vi "UHR-Fleezers Control (host) -Mau_stepping_gamma.vi"(0 "Tab Control":T5(tab)) -> ()   [LabVIEW 2013] (continued)
  n71 = local write "Update Count (MCL)"(w101) -> ()
  n72 = local write "Total Counts (ticks)"(w101) -> ()
  n73 = xnode "Invoke Method"("FPGA VI Reference In"=w218) -> ("FPGA VI Reference Out"=w120:T19, "error out"=w139:errorcluster)  [unwired: 1 in]
  n74 = local write "Ave. Period (s)"(w170) -> ()
  n75 = property on="2D or 1D Scan" class="Bool (strict)"("Val(Sgnl)"=w122) -> ()  [unwired: 2 in, 2 out]
  n76 = xnode "Read/Write Control"("FPGA VI Reference In"=w119, "error in"=w139, "ai count"="AI Count (ticks)", "Interlace ON/OFF"=w104, "Number Interlace Cycles"=w103, "AI1 Sets to FIFO"=w233, "FB On/Off Set 1"=w232, "FB On/Off Set 2"=w231, "Interlace Off Parameters"=w102, "FB Setpoint Set 1"=w223, "FB Setpoint Set 2"=w222, "FB Gains Set 1"=w220, "FB Gains Set 2"=w219, "FB output range 1"=w121, "FB output range 2"=w121, "Cycles per step"=w204, "Scan BD"=w216, "Number of scans"=w200, "Scan steps"=w205, "Scan freq.  increment"=w206, "AO1"=w188, "AO2"=w187, "Scan freq.  increment (MCL)"=w181, "Scan steps (MCL)"=w180, "Cycles per step (MCL)"=w179, "Number of scans (MCL)"=w178, "MCL count"=w101, "Cont. Scan (MCL)"=w177, "MCL Scan Axis"=w171, "1D or 2D Scan?"=w122, "N of AI1 Int Acq Sets"=w161, "Freq or Amp switch first"="Freq or Amp switch first", "Freq switch delay"="Freq switch delay", "Amp switch delay"="Amp switch delay", "Swap F1 and F2"="Swap F1 and F2", "APD Acq Rate Count"=w127, "APD to FIFO"=FALSE, "APD Gate Operating Mode"="APD Gate", "APD Gate ON Count"="APD Gate ON Count", "APD Gate OFF Count"="APD Gate OFF Count", "Invert APD Gate"="Invert APD Gate", "DIO count 1 (ticks)"="DIO count 1 (ticks)", "DIO count 2 (ticks)"="DIO count 2 (ticks)", "DIO count 3 (ticks)"="DIO count 3 (ticks)", "APD 1 AO scale factor"="APD 1 AO Mult.", "APD 2 AO scale factor"="APD 2 AO Mult.") -> ("FPGA VI Reference Out"=w96:T19, "error out"=w98:errorcluster)  [unwired: 1 in]
  n77 = local read "Green Laser ON/Interlacing"() -> (w99:bool)
  n78 = local read "Green laser mode"() -> (w100:enum32{"Laser ON", "Laser OFF", "Interlace"})
  n79 = local read "GI Frequency, OFF count"() -> (w92:u32)
  n80 = local read "GI Frequency, ON count"() -> (w91:u32)
  n81 = Multiply(x="Current When FB OFF (%)", y=655.35) -> (x*y=w82:dbl)
  n82 = local read "Green FB Count"() -> (w90:u32)
  n83 = Multiply(x="Green FB Setpoint (mV)", y=3.2767) -> (x*y=w79:dbl)
  n84 = To Unsigned Word Integer(number=w82) -> (unsigned 16bit integer=w80:u16)
  n85 = local read "Invert GI"() -> (w94:bool)
  n86 = To Word Integer(number=w79) -> (16bit integer=w77:i16)
  n87 = case shown="True" w99 {
    tunnel: w100 -> [_ w253]
    tunnel: [enum32{"Laser ON", "Laser OFF", "Interlace"}."Laser OFF" ("Green laser mode") w253] -> w93
    frame False {
    }
    frame True {
    }
  }
  n88 = local read "Trap Pos. AI1 X Pre-scale"() -> (w48:u16)
  n89 = local read "Trap Pos FB Monitor\nT1 or T2"() -> (w55:bool)
  n90 = local read "Trap Pos FB Int Count"() -> (w43:u16)
  n91 = local read "Trap Pos FB Negate Action"() -> (w54:bool)
  n92 = local read "Trap Pos. FB Offset Factor"() -> (w53:i64)
  n93 = local read "Trap Pos. FB Mult Factor"() -> (w52:i64)
  n94 = local read "Trap Pos. FB Gains"() -> (w50:T11)
  n95 = local read "Trap Pos. FB Range"() -> (w51:T12)
  n96 = xnode "Read/Write Control"("FPGA VI Reference In"=w96, "error in"=w98, "Green interlace ON count 2"=w91, "Green interlace OFF count 2"=w92, "Invert GI 2"=w94, "Operating Mode 2"=w93, "Green FB Gains"="Green FB Gains", "Green FB Setpoint"=w77, "Green FB On/Off"="Green FB On/Off", "Current Out"=w80, "Green int current ON count adj"="Green int current ON count adj", "Green FB Count"=w90, "Operating Mode"=w93, "Green interlace OFF count"=w92, "Green interlace ON count"=w91, "Invert GI"=w94, "Trap Pos FB Monitor T1 or T2"=w55, "Trap Pos FB Negate Action"=w54, "Trap Pos. FB Offset Factor"=w53, "Trap Pos. FB Mult Factor"=w52, "Trap Pos. FB Range"=w51, "Trap Pos. FB Gains"=w50, "Force feedback"=FALSE, "AI1 X Scale"=w48, "Trap Pos to FIFO"=TRUE, "Trap Pos FB Int Count"=w43) -> ("FPGA VI Reference Out"=w95:T19, "error out"=w97:errorcluster)
  n97 = xnode "Invoke Method"("FPGA VI Reference In"=w95, "error in"=w97, "Requested Depth"="Trap AI FIFO Depth") -> ("FPGA VI Reference Out"=w58:T19, "error out"=w57:errorcluster)  [unwired: 1 out]
  n98 = xnode "Invoke Method"("FPGA VI Reference In"=w58, "error in"=w57, "Requested Depth"="Trap Position FIFO Depth") -> ("FPGA VI Reference Out"=w45:T19, "error out"=w44:errorcluster)  [unwired: 1 out]
  n99 = flat-sequence {
    tunnel: w120 -> [w258]
    tunnel: [w258] -> w119
    tunnel: [w257] -> w118
    tunnel: [w256] -> w117
    tunnel: [w254] -> w115
    tunnel: [w255] -> w116
    frame #0 {
      w255 = T16 {"Minimum"=50.0, "Maximum"=100.0, "Increment"=1.0} ("Min Max Inc")
      w254 = T16 {"Minimum"=0.0, "Maximum"=75.0, "Increment"=1.0} ("Data Entry Limits")
      w257 = T16 {"Minimum"=50.0, "Maximum"=100.0, "Increment"=1.0} ("Min Max Inc")
      w256 = T16 {"Minimum"=0.0, "Maximum"=75.0, "Increment"=1.0} ("Data Entry Limits")
      n100 = property on="BD 2 Frequency 1 (MHz)" class="DigNum (strict)"("Data Range"=w255) -> ()  [unwired: 2 in, 2 out]
      n101 = property on="BD 2 Frequency 3 (MHz)" class="DigNum (strict)"("Data Range"=w255) -> ()  [unwired: 2 in, 2 out]
      n102 = property on="BD 2 Frequency 2 (MHz)" class="DigNum (strict)"("Data Range"=w255) -> ()  [unwired: 2 in, 2 out]
      n103 = property on="BD 1 Frequency 1 (MHz)" class="DigNum (strict)"("Data Range"=w257) -> ()  [unwired: 2 in, 2 out]
      n104 = property on="BD 1 Frequency 2 (MHz)" class="DigNum (strict)"("Data Range"=w257) -> ()  [unwired: 2 in, 2 out]
      n105 = property on="BD 1 Frequency 3 (MHz)" class="DigNum (strict)"("Data Range"=w257) -> ()  [unwired: 2 in, 2 out]
      n106 = property on="BD 2 Amplitude 1 (%)" class="DigNum (strict)"("Data Range"=w254) -> ()  [unwired: 2 in, 2 out]
      n107 = property on="BD 2 Amplitude 2 (%)" class="DigNum (strict)"("Data Range"=w254) -> ()  [unwired: 2 in, 2 out]
      n108 = property on="BD 2 Amplitude 3 (%)" class="DigNum (strict)"("Data Range"=w254) -> ()  [unwired: 2 in, 2 out]
      n109 = property on="BD 1 Amplitude 3 (%)" class="DigNum (strict)"("Data Range"=w256) -> ()  [unwired: 2 in, 2 out]
      n110 = property on="BD 1 Amplitude 2 (%)" class="DigNum (strict)"("Data Range"=w256) -> ()  [unwired: 2 in, 2 out]
      n111 = property on="BD 1 Amplitude 1 (%)" class="DigNum (strict)"("Data Range"=w256) -> ()  [unwired: 2 in, 2 out]
      "X RF Frequency Limits (MHz)" <- w257
      "X RF Amplitude Limits (%)" <- w256
      "Y RF Amplitude Limits (%)" <- w254
      "Y RF Frequency Limits (MHz)" <- w255
    }
  }
  n112 = xnode "Invoke Method"("FPGA VI Reference In"=w45, "error in"=w44) -> ("FPGA VI Reference Out"=w22:T19, "error out"=w21:errorcluster)  [unwired: 1 in]
  n113 = flat-sequence "Initial FPGA Loop Relative Phase Adjustment" {
    tunnel: "Initial Phase Adjustment (APD 2 Gate)" -> [w260]
    tunnel: "Initial Phase Adjustment (GI) 2" -> [w261]
    tunnel: "Initial Phase Adj. (MCL)" -> [w262]
    tunnel: w21 -> [w263]
    tunnel: w22 -> [w264]
    tunnel: "Initial Phase Adjustment (GI)" -> [w265]
    tunnel: "Initial Phase Adjustment (AI1)" -> [w266]
    tunnel: [w266] -> w31
    tunnel: [w265] -> w30
    tunnel: [w264] -> w29
    tunnel: [w263] -> w28
    tunnel: [w262] -> w27
    tunnel: [w261] -> w26
    tunnel: [w260] -> w25
    tunnel: [w278] -> w145
    tunnel: [w272] -> w143
    tunnel: "Initial Phase Adjustment (APD Acq)" -> [w271]
    tunnel: "Initial Phase Adjustment (APD 1 Gate)" -> [w270]
    tunnel: "Initial Phase Adjustment (Green FB)" -> [w269]
    tunnel: w31 -> [w277]
    tunnel: w30 -> [w276]
    tunnel: w29 -> [w275]
    tunnel: w28 -> [w274]
    tunnel: w27 -> [w273]
    tunnel: w26 -> [w268]
    tunnel: w25 -> [w267]
    tunnel: w145 -> [w280]
    tunnel: [w281] -> w144
    tunnel: w143 -> [w281]
    tunnel: [w280] -> w142
    tunnel: w144 -> [w284]
    tunnel: w142 -> [w283]
    tunnel: [w286] -> w141
    tunnel: [w285] -> w140
    tunnel: [w288] -> w20
    tunnel: [w289] -> w23
    tunnel: w141 -> [w289]
    tunnel: w140 -> [w288]
    frame #0 {
      n114 = Wait (ms)(milliseconds to wait=u32 1000) -> ()  [unwired: 1 out]
    }
    frame #1 {
      n115 = xnode "Read/Write Control"("FPGA VI Reference In"=w275, "error in"=w274, "Phase count adjustment"=w277, "Phase count adjustment (GI)"=w276, "Phase count adjustment (MCL)"=w273, "Phase Count Adjustment (APD Acq)"=w271, "Phase count adjustment (APD 1 Gate)"=w270, "Phase count adjustment (APD 2 Gate)"=w267, "Phase count adjustment (Green FB)"=w269, "Phase count adjustment (GI) 2"=w268) -> ("FPGA VI Reference Out"=w272:T19, "error out"=w278:errorcluster)
    }
    frame #2 {
      n116 = Wait (ms)(milliseconds to wait=u32 1000) -> ()  [unwired: 1 out]
    }
    frame #3 {
      w282 = TRUE
      n117 = xnode "Read/Write Control"("FPGA VI Reference In"=w284, "error in"=w283, "+ phase"=w282, "+ phase (GI)"=w282, "+ phase (MCL)"=w282, "+ phase (APD Acq)"=w282, "+ phase (APD 1 Gate)"=w282, "+ phase (APD 2 Gate)"=w282, "+ phase (Green FB)"=w282, "+ phase (GI) 2"=w282) -> ("FPGA VI Reference Out"=w285:T19, "error out"=w286:errorcluster)
    }
    frame #4 {
      n118 = Wait (ms)(milliseconds to wait=u32 1000) -> ()  [unwired: 1 out]
    }
  }
  n119 = local read "Phase adj. (Green FB)"() -> (w113:i16)
  n120 = local read "Phase adj. (GI) 2"() -> (w83:i16)
  n121 = local read "Phase adjust (MCL)"() -> (w172:i16)
  n122 = local read "Phase adj. (AI1)"() -> (w174:i16)
  n123 = local read "Phase adj. (GI)"() -> (w173:i16)
  n124 = xnode "Read/Write Control"("FPGA VI Reference In"=w20, "error in"=w23, "Phase count adjustment"=w174, "Phase count adjustment (GI)"=w173, "Phase count adjustment (MCL)"=w172, "Phase Count Adjustment (APD Acq)"="Phase Adj. (APD Acq)", "Phase count adjustment (APD 1 Gate)"="Phase Adj. (APD 1 Gate)", "Phase count adjustment (APD 2 Gate)"="Phase Adj. (APD 2 Gate)", "Phase count adjustment (Green FB)"=w113, "Phase count adjustment (GI) 2"=w83) -> ("FPGA VI Reference Out"=w19:T19, "error out"=w18:errorcluster)
  n125 = call "Initialize RF boards - interlace 3.vi"("error in"=w18, "FPGA VI Reference In"=w19) -> ("FPGA VI Reference Out"=w150:T19)  [unwired: 1 out]
  n126 = call "set RF board frequency - interlace.vi"("Board 2 Frequency Limits"=w116, "Board 1 Frequency Limits"=w118, "FPGA VI Reference In"=w150, "Board 2 Frequency 3 (MHz)"="BD 2 Frequency 3 (MHz)", "Board 1 Frequency 3 (MHz)"="BD 1 Frequency 3 (MHz)", "Board 2 Frequency 2 (MHz)"="BD 2 Frequency 2 (MHz)", "Board 2 Frequency 1 (MHz)"="BD 2 Frequency 1 (MHz)", "Board 1 Frequency 2 (MHz)"="BD 1 Frequency 2 (MHz)", "Board 1 Frequency 1  (MHz)"="BD 1 Frequency 1 (MHz)") -> ("error out"=w244:errorcluster, "FPGA VI Reference Out"=w245:T19)  [unwired: 1 in]
  n127 = call "set RF board amplitude - interlace.vi"("Board 2 Amplitude Limits"=w115, "Board 1 Amplitude Limits"=w117, "error in"=w244, "FPGA VI Reference In"=w245, "Board 2 Amplitude 3 (%)"="BD 2 Amplitude 3 (%)", "Board 1 Amplitude 3 (%)"="BD 1 Amplitude 3 (%)", "Board 2 Amplitude 2 (%)"="BD 2 Amplitude 2 (%)", "Board 2 Amplitude 1 (%)"="BD 2 Amplitude 1 (%)", "Board 1 Amplitude 2 (%)"="BD 1 Amplitude 2 (%)", "Board 1 Amplitude 1 (%)"="BD 1 Amplitude 1 (%)") -> ("error out"=w16:errorcluster, "FPGA VI Reference Out"=w17:T19)
  n128 = flat-sequence {
    tunnel: w17 -> [w298]
    tunnel: w16 -> [w297]
    tunnel: [w296] -> w237
    tunnel: [w295] -> w236
    tunnel: [w302] -> w235
    tunnel: w237 -> [w302]
    tunnel: [w301] -> w234
    tunnel: w236 -> [w301]
    tunnel: w235 -> [w311]
    tunnel: w234 -> [w310]
    tunnel: [w309] -> w12
    tunnel: [w304] -> w11
    tunnel: [w314] -> w40
    tunnel: [w318] -> w24
    tunnel: w12 -> [w318]
    tunnel: w11 -> [w313]
    frame #0 {
      n129 = local read "Trap 1 (ON/OFF)"() -> (w290:bool)
      n130 = xnode "Read/Write Control"("FPGA VI Reference In"=w298, "error in"=w297, "Direct RF Box  Communication"=FALSE) -> ("FPGA VI Reference Out"=w296:T19, "error out"=w295:errorcluster)
      n131 = local write "Saving..."(FALSE ("Saving Data")) -> ()
      n132 = local write "Stop All"(FALSE ("Stop All")) -> ()
      n133 = local write "Index"(1.0 ("Index")) -> ()
      n134 = property on="Trap 1 ON" class="Bool (strict)"("Value"=w290) -> ()  [unwired: 2 in, 2 out]
      "Manipulating Trap" <- FALSE ("Manipulating Trap")
    }
    frame #1 {
      n135 = local read "Trap 2 (ON/OFF)"() -> (w300:bool)
      n136 = Wait (ms)(milliseconds to wait=u32 50) -> ()  [unwired: 1 out]
      n137 = property on="Trap 2 ON" class="Bool (strict)"("Val(Sgnl)"=w300) -> ()  [unwired: 2 in, 2 out]
    }
    frame #2 {
      n138 = local read "Scan Range (nm)"() -> (w305:dbl)
      n139 = xnode "Read/Write Control"("FPGA VI Reference In"=w311, "error in"=w310, "FPGA Controls  RF Box"=TRUE ("Direct RF Box  Communication")) -> ("FPGA VI Reference Out"=w309:T19, "error out"=w304:errorcluster)
      n140 = call "Update messages.vi"("Message to add"="UHR-Fleezers ready.", "Old message string"="") -> ("New message string"=w308:string)
      n141 = local write "Messages"(w308) -> ()
      n142 = property on="Scan Range (nm)" class="DigNum (strict)"("Val(Sgnl)"=w305) -> ()  [unwired: 2 in, 2 out]
    }
    frame #3 {
      n143 = call "hamilton_controller.vi"("error in"=w313, "action"=T20."CONNECT") -> ("error out"=w315:errorcluster)  [unwired: 9 in]
      n144 = call "hamilton_controller.vi"("error in"=w315, "action"=T20."INITIALIZE VALVES") -> ("error out"=w314:errorcluster)  [unwired: 9 in]
    }
  }
  n145 = Subtract(x="BD 1 Frequency 1 (MHz)", y="BD 1 Frequency 2 (MHz)") -> (x-y=w160:dbl)
  n146 = Subtract(x="BD 2 Frequency 1 (MHz)", y="BD 2 Frequency 2 (MHz)") -> (x-y=w159:dbl)
  n147 = Square(x=w159) -> (x^2=w157:dbl)
  n148 = Square(x=w160) -> (x^2=w158:dbl)
  n149 = Add(x=w158, y=w157) -> (x+y=w156:dbl)
  n150 = Square Root(x=w156) -> (sqrt(x)=w155:dbl)
  n151 = local write "Trap Delta (MHz)"(w155) -> ()
  n152 = call "IMAQ Create"("Image Name"="APD 1 Image", "Image Type"=w64) -> ("New Image"=w63:T3)  [unwired: 3 in, 1 out]
  n153 = call "IMAQ Create"("Image Name"="APD 2 Image", "Image Type"=w64) -> ("New Image"=w62:T3)  [unwired: 3 in, 1 out]
  n154 = call "IMAQ Create"("Image Name"="Det. X Image", "Image Type"=w64) -> ("New Image"=w61:T3)  [unwired: 3 in, 1 out]
  n155 = call "IMAQ Create"("Image Name"="Det. Y Image", "Image Type"=w64) -> ("New Image"=w60:T3)  [unwired: 3 in, 1 out]
  n156 = Bundle("New Image"=w63, "New Image"=w62, "New Image"=w61, "New Image"=w60) -> (w59:T21)  [unwired: 1 in]
  n157 = Current VI's Path() -> (path=w1:path)
  n158 = Concatenate Strings("N.D.", "\r\n") -> (w5:string)
  n159 = Strip Path(path=w1) -> (stripped path=w2:path)  [unwired: 1 out]
  n160 = Initialize Array(w5, 4, 3) -> (w8:string[][])
  n161 = Build Path(base path=w2, name or relative path="Locations.txt") -> (appended path=→"Location path":path)
  n162 = local write "Location Matrix"(w8) -> ()
  n163 = while {
    stop <- w319 stop-if-true
    n164 = event shown="[0] Timeout" {
      selector: _ -> [_ _ _ _ _ _ _ _]
      dyn-events: _ -> [_ _ _ _ _ _ _ _]
      timeout: 10 -> [_ _ _ _ _ _ _ _]
      tunnel: [FALSE _ TRUE _ _ _ _ _] -> w319
      event Timeout {
        # "Change the trajectory mode to Jog"
        # "Query and display stage positions"
        # "Setting ESP300 left and right limits for Z-axis, input in mm"
        # "Display Selected Location"
        n165 = event-data() -> ()  [unwired: 1 in, 2 out]
        n166 = local read "Capture Locations"() -> (w344:i32)
        n167 = local read "Location Matrix"() -> (w345:string[][])
        n168 = Concatenate Strings("1TP;\n2TP;\n3TP;\n1MD?;\n2MD?;\n3MD?" ("Substring"), "\r") -> (w328:string)
        n169 = local read "ESP Port"() -> (w331:refnum<visa-resource-name>)
        n170 = Index Array(array=w345, index (row)=w344) -> (element=w343:string[])  [unwired: 1 in]
        n171 = local read "ESP Port"() -> (w340:refnum<visa-resource-name>)
        n172 = VISA Write(VISA resource name=w331, write buffer=w328, error in (no error)="error in") -> (VISA resource name out=w329:refnum<visa-resource-name>, error out=w327:errorcluster)  [unwired: 1 out]
        n173 = Concatenate Strings("3SL" ("Substring"), "ESP ZL-Limit", ";3SR", "ESP ZR-Limit", "\r") -> (w339:string)
        n174 = Array To Cluster(array=w343) -> (cluster=w342:T22)
        n175 = case shown="True" TRUE ("Case Constant\n(See Context Help)") {
          tunnel: w329 -> [_ w383]
          tunnel: w327 -> [w364 w382]
          tunnel: [w364 w366] -> w333
          frame False {
          }
          frame True {
            w376 = u16 10 items=["1.0"=10, "1.5"=15, "2.0"=20] ("Serial Settings:Stop Bits")
            w377 = u16 0 items=["None", "Odd", "Even", "Mark", "Space"] ("Serial Settings:Parity")
            n176 = property class="Instr"(reference=w383, error in=w382, "Baud"=u32 921600 ("Serial Settings:Baud Rate"), "Data Bits"=u16 8 ("Serial Settings:Data Bits"), "Parity"=w377, "Stop Bits"=w376) -> (reference out=w381:refnum<visa-resource-name>, error out=w380:errorcluster, "Bytes at Port"=w365:u32)
            n177 = Wait (ms)(milliseconds to wait=u32 10) -> ()  [unwired: 1 out]
            n178 = VISA Read(VISA resource name=w381, byte count=w365, error in (no error)=w380) -> (VISA resource name out=w389:refnum<visa-resource-name>, read buffer=→"X Pos":string, error out=w390:errorcluster)  [unwired: 1 out]
            n179 = VISA Read(VISA resource name=w389, byte count=w365, error in (no error)=w390) -> (VISA resource name out=w387:refnum<visa-resource-name>, read buffer=→"Y Pos":string, error out=w388:errorcluster)  [unwired: 1 out]
            n180 = VISA Read(VISA resource name=w387, byte count=w365, error in (no error)=w388) -> (VISA resource name out=w375:refnum<visa-resource-name>, read buffer=→"Z Pos Pos":string, error out=w374:errorcluster)  [unwired: 1 out]
            n181 = VISA Read(VISA resource name=w375, byte count=w365, error in (no error)=w374) -> (VISA resource name out=w371:refnum<visa-resource-name>, read buffer=→"X Motion":string, error out=w372:errorcluster)  [unwired: 1 out]
            n182 = VISA Read(VISA resource name=w371, byte count=w365, error in (no error)=w372) -> (VISA resource name out=w370:refnum<visa-resource-name>, read buffer=→"Y Motion":string, error out=w368:errorcluster)  [unwired: 1 out]
            n183 = VISA Read(VISA resource name=w370, byte count=w365, error in (no error)=w368) -> (read buffer=→"Z motion":string, error out=w366:errorcluster)  [unwired: 2 out]
          }
        }
        "error out" <- w333
        n184 = VISA Write(VISA resource name=w340, write buffer=w339) -> ()  [unwired: 1 in, 3 out]
        n185 = local write item#485(w342) -> ()
        n186 = disable-structure shown="Disabled" {
          frame Disabled {
            # "Change Low Jog Velocity"
            # "Change High Jog Velocity"
            n187 = Concatenate Strings("1JH" ("Substring"), "Axis 1", "2JH" ("Substring"), "Axis 2", "3JH" ("Substring"), "Axis 3", "\r") -> (w363:string)
            n188 = local read "ESP Port"() -> (w362:refnum<visa-resource-name>)
            n189 = VISA Write(VISA resource name=w362, write buffer=w363) -> ()  [unwired: 1 in, 3 out]
            n190 = Concatenate Strings("1JW" ("Substring"), "Axis 1", "2JW" ("Substring"), "Axis 2", "3JW" ("Substring"), "Axis 3", "\r") -> (w354:string)
            n191 = local read "ESP Port"() -> (w353:refnum<visa-resource-name>)
            n192 = VISA Write(VISA resource name=w353, write buffer=w354) -> ()  [unwired: 1 in, 3 out]
          }
          frame Enabled {
          }
        }
        n193 = local read "ESP Port"() -> (w321:refnum<visa-resource-name>)
        n194 = Concatenate Strings("1TJ3;\n2TJ3;\n3TJ3" ("Substring"), "\r") -> (w322:string)
        n195 = VISA Write(VISA resource name=w321, write buffer=w322) -> ()  [unwired: 1 in, 3 out]
      }
      event "Goto Top (F6)": Value Change {
        n196 = event-data() -> ()  [unwired: 1 in, 5 out]
        n197 = stacked-sequence {
          frame #0 {
            # "stop motions of all axes before going to avoid reversing of direction"
            n198 = local read "ESP Port"() -> (w395:refnum<visa-resource-name>)
            n199 = Concatenate Strings("ST" ("Substring"), "\r") -> (w392:string)
            n200 = VISA Write(VISA resource name=w395, write buffer=w392) -> ()  [unwired: 1 in, 3 out]
          }
          frame #1 {
            n201 = Wait (ms)(milliseconds to wait=u32 50) -> ()  [unwired: 1 out]
          }
          frame #2 {
            # "Change the trajectory mode to Trapezoidal"
            n202 = local read "ESP Port"() -> (w400:refnum<visa-resource-name>)
            n203 = Concatenate Strings("1TJ1;\n2TJ1;\n3TJ1" ("Substring"), "\r") -> (w397:string)
            n204 = VISA Write(VISA resource name=w400, write buffer=w397) -> ()  [unwired: 1 in, 3 out]
          }
          frame #3 {
            # "Go to Top Dispensor"
            n205 = local read "Location Matrix"() -> (w412:string[][])
            n206 = Index Array(array=w412, index (row)=0) -> (element=w408:string[])  [unwired: 1 in]
            n207 = Decimate 1D Array(w408) -> (w406:string[], w404:string[], w402:string[])
            n208 = local read "ESP Port"() -> (w409:refnum<visa-resource-name>)
            n209 = Concatenate Strings("1PA" ("Substring"), w406, "2PA" ("Substring"), w404, "3PA" ("Substring"), w402, "\r") -> (w410:string)
            n210 = VISA Write(VISA resource name=w409, write buffer=w410) -> ()  [unwired: 1 in, 3 out]
          }
          frame #4 {
            n211 = Wait (ms)(milliseconds to wait=u32 100) -> ()  [unwired: 1 out]
          }
          frame #5 {
            # "Change the trajectory mode to Jog"
            n212 = local read "ESP Port"() -> (w417:refnum<visa-resource-name>)
            n213 = Concatenate Strings("1TJ3;\n2TJ3;\n3TJ3" ("Substring"), "\r") -> (w414:string)
            n214 = VISA Write(VISA resource name=w417, write buffer=w414) -> ()  [unwired: 1 in, 3 out]
          }
        }
      }
      event "Stop All": Mouse Down {
        n215 = event-data() -> ()  [unwired: 1 in, 5 out]
      }
      event "Goto Exp (F8)": Value Change {
        n216 = event-data() -> ()  [unwired: 1 in, 5 out]
        n217 = stacked-sequence {
          frame #0 {
            # "stop motions of all axes before going to avoid reversing of direction"
            n218 = local read "ESP Port"() -> (w422:refnum<visa-resource-name>)
            n219 = Concatenate Strings("ST" ("Substring"), "\r") -> (w419:string)
            n220 = VISA Write(VISA resource name=w422, write buffer=w419) -> ()  [unwired: 1 in, 3 out]
          }
          frame #1 {
            n221 = Wait (ms)(milliseconds to wait=u32 50) -> ()  [unwired: 1 out]
          }
          frame #2 {
            # "Change the trajectory mode to Trapezoidal"
            n222 = local read "ESP Port"() -> (w427:refnum<visa-resource-name>)
            n223 = Concatenate Strings("1TJ1;\n2TJ1;\n3TJ1" ("Substring"), "\r") -> (w424:string)
            n224 = VISA Write(VISA resource name=w427, write buffer=w424) -> ()  [unwired: 1 in, 3 out]
          }
          frame #3 {
            # "Go to Experimental"
            n225 = local read "Location Matrix"() -> (w439:string[][])
            n226 = Index Array(array=w439, index (row)=2) -> (element=w435:string[])  [unwired: 1 in]
            n227 = Decimate 1D Array(w435) -> (w433:string[], w431:string[], w429:string[])
            n228 = Concatenate Strings("1PA" ("Substring"), w433, "2PA" ("Substring"), w431, "3PA" ("Substring"), w429, "\r") -> (w437:string)
            n229 = local read "ESP Port"() -> (w436:refnum<visa-resource-name>)
            n230 = VISA Write(VISA resource name=w436, write buffer=w437) -> ()  [unwired: 1 in, 3 out]
          }
          frame #4 {
            n231 = Wait (ms)(milliseconds to wait=u32 200) -> ()  [unwired: 1 out]
          }
          frame #5 {
            # "Change the trajectory mode to Jog"
            n232 = local read "ESP Port"() -> (w441:refnum<visa-resource-name>)
            n233 = Concatenate Strings("1TJ3;\n2TJ3;\n3TJ3" ("Substring"), "\r") -> (w444:string)
            n234 = VISA Write(VISA resource name=w441, write buffer=w444) -> ()  [unwired: 1 in, 3 out]
          }
        }
      }
      event "Goto Bottom (F7)": Value Change {
        n235 = event-data() -> ()  [unwired: 1 in, 5 out]
        n236 = stacked-sequence {
          frame #0 {
            # "stop motions of all axes before going to avoid reversing of direction"
            n237 = local read "ESP Port"() -> (w448:refnum<visa-resource-name>)
            n238 = Concatenate Strings("ST" ("Substring"), "\r") -> (w445:string)
            n239 = VISA Write(VISA resource name=w448, write buffer=w445) -> ()  [unwired: 1 in, 3 out]
          }
          frame #1 {
            n240 = Wait (ms)(milliseconds to wait=u32 50) -> ()  [unwired: 1 out]
          }
          frame #2 {
            # "Change the trajectory mode to Trapezoidal"
            n241 = local read "ESP Port"() -> (w453:refnum<visa-resource-name>)
            n242 = Concatenate Strings("1TJ1;\n2TJ1;\n3TJ1" ("Substring"), "\r") -> (w450:string)
            n243 = VISA Write(VISA resource name=w453, write buffer=w450) -> ()  [unwired: 1 in, 3 out]
          }
